vi "Is Pre Amp Gain Available.vi"(6 "status":i32, 7 "pa":i32, 8 "error in (no error)":errorcluster, 9 "index":i32, 10 "amplifier":i32, 11 "channel":i32) -> (0 "error out":errorcluster, 3 "function return":u32, 4 "status out":i32)   [LabVIEW 2014, in "atmcd32d.lvlib"]
doc: "unsigned int WINAPI IsPreAmpGainAvailable(int channel, int amplifier, int index, int pa, int * status);"
uses:
  atmcd32d.lvlib
  atmcd32d.dll
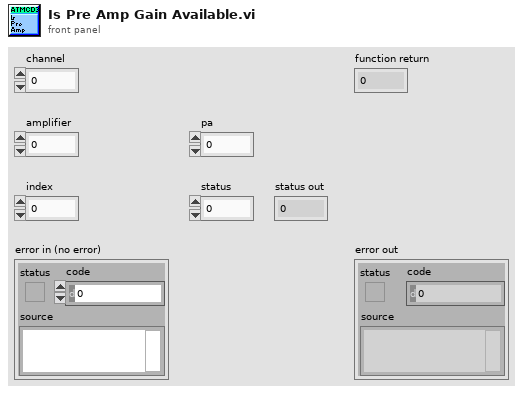
[diagram p1: front panel]
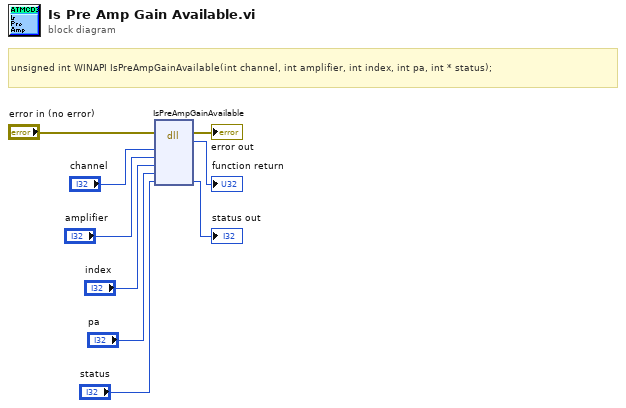
[diagram p0: block diagram]
diagram:
  # "unsigned int WINAPI IsPreAmpGainAvailable(int channel, int amplifier, int index, int pa, int * status);"
  n1 = dll-call lib="C:/Users/Bakir/Documents/Lambda2-Testing/lib/Andorlib/atmcd32d.*" fn="IsPreAmpGainAvailable"(error in="error in (no error)", "channel"="channel", "amplifier"="amplifier", "index"="index", "pa"="pa", "status"="status") -> (error out=→"error out":errorcluster, →"function return":u32, "status"=→"status out":i32)  [unwired: 6 in, 1 out]
